vi "offload product.vi"   [LabVIEW 2023]
types:
  T1 = enum16{"plate1", "plate2", "plate3", "rinse", "seat"}
  T2 = enum16{"Initialize", "Absolute Position", "Relative Pickup", "Relative Dispense", "Swich valve", "Bypass"}
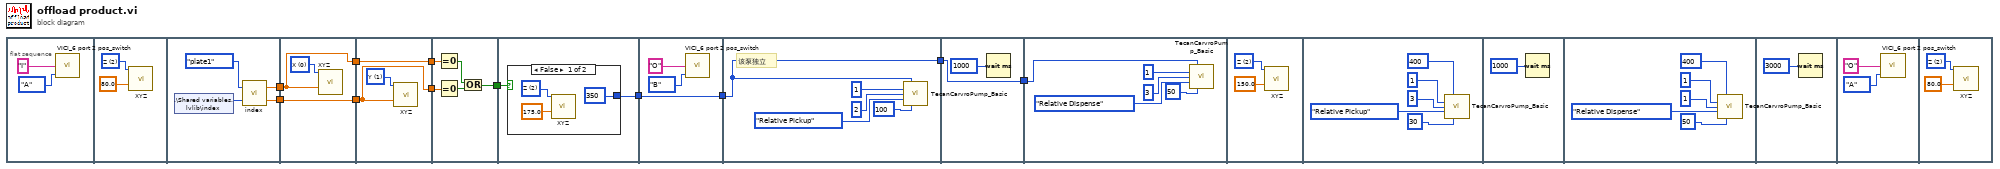
[diagram p0: block diagram]
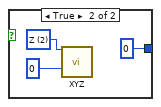
[diagram p2: hidden frame]
diagram:
  n1 = flat-sequence {
    tunnel: [w19] -> w11
    tunnel: [w18] -> w9
    tunnel: w11 -> [w20]
    tunnel: [w21] -> w10
    tunnel: w9 -> [w21]
    tunnel: [w20] -> w7
    tunnel: w10 -> [w23]
    tunnel: [w24] -> w8
    tunnel: w7 -> [w24]
    tunnel: [w23] -> w6
    tunnel: w8 -> [w30]
    tunnel: w6 -> [w29]
    tunnel: [w26] -> w5
    tunnel: w5 -> [w32]
    tunnel: [w31] -> w3
    tunnel: [w39] -> w4
    tunnel: w3 -> [w39]
    tunnel: w4 -> [w42]
    tunnel: [w42] -> w2
    tunnel: [w47] -> w1
    tunnel: w2 -> [w47]
    tunnel: w1 -> [w49]
    frame #0 {
      n2 = call "VICI_6 port 2 pos_switch.vi"("Switch to position (A/B)"=enum16{"A", "B"}."A", "Valve ID"="I") -> ()  [unwired: 2 in, 1 out]
    }
    frame #1 {
      w15 = u16 2 items=["X", "Y", "Z"] ("AXIS")
      n3 = call "XYZ.vi"("AXIS"=w15, "Set location (mm)"=80.0) -> ()  [unwired: 9 in, 5 out]
    }
    frame #2 {
      n4 = shared-variable ".\\Shared variables.lvlib\\index"() -> (w16:i8)  [unwired: 1 in, 1 out]
      n5 = call "index.vi"("index"=w16, "where"=T1."plate1") -> ("Y"=w18:dbl, "X"=w19:dbl)
    }
    frame #3 {
      w22 = u16 0 items=["X", "Y", "Z"] ("AXIS")
      n6 = call "XYZ.vi"("AXIS"=w22, "Set location (mm)"=w20) -> ()  [unwired: 9 in, 5 out]
    }
    frame #4 {
      w25 = u16 1 items=["X", "Y", "Z"] ("AXIS")
      n7 = call "XYZ.vi"("AXIS"=w25, "Set location (mm)"=w23) -> ()  [unwired: 9 in, 5 out]
    }
    frame #5 {
      n8 = Equal To 0?(x=w30) -> (x = 0?=w28:bool)
      n9 = Equal To 0?(x=w29) -> (x = 0?=w27:bool)
      n10 = Or(x=w28, y=w27) -> (x .or. y?=w26:bool)
    }
    frame #6 {
      n11 = case shown="False" w32 {
        tunnel: [u16 350 ("Volume (μL)") u16 0 ("Volume (μL)")] -> w31
        frame False {
          w35 = u16 2 items=["X", "Y", "Z"] ("AXIS")
          n12 = call "XYZ.vi"("AXIS"=w35, "Set location (mm)"=175.0) -> ()  [unwired: 9 in, 5 out]
        }
        frame True {
          w37 = u16 2 items=["X", "Y", "Z"] ("AXIS")
          n13 = call "XYZ.vi"("AXIS"=w37, "Set location (mm)"=0) -> ()  [unwired: 9 in, 5 out]
        }
      }
    }
    frame #7 {
      n14 = call "VICI_6 port 2 pos_switch.vi"("Switch to position (A/B)"=enum16{"A", "B"}."B", "Valve ID"="O") -> ()  [unwired: 2 in, 1 out]
    }
    frame #8 {
      # "该泵独立"
      n15 = call "TecanCarvroPump_Basic.vi"("Volume (μL)"=w42, "TecanPump address"=u8 1, "Valve"=u8 2, "Mode"=T2."Relative Pickup", "Speed (μL/s)"=u16 100) -> ()  [unwired: 10 in, 1 out]
    }
    frame #9 {
      n16 = Wait (ms)(milliseconds to wait=u32 1000) -> ()  [unwired: 1 out]
    }
    frame #10 {
      n17 = call "TecanCarvroPump_Basic.vi"("Volume (μL)"=w49, "TecanPump address"=u8 1, "Valve"=u8 3, "Mode"=T2."Relative Dispense", "Speed (μL/s)"=u16 50) -> ()  [unwired: 10 in, 1 out]
    }
    frame #11 {
      w55 = u16 2 items=["X", "Y", "Z"] ("AXIS")
      n18 = call "XYZ.vi"("AXIS"=w55, "Set location (mm)"=150.0) -> ()  [unwired: 9 in, 5 out]
    }
    frame #12 {
      n19 = call "TecanCarvroPump_Basic.vi"("Volume (μL)"=u16 400, "TecanPump address"=u8 1, "Valve"=u8 3, "Mode"=T2."Relative Pickup", "Speed (μL/s)"=u16 30) -> ()  [unwired: 10 in, 1 out]
    }
    frame #13 {
      n20 = Wait (ms)(milliseconds to wait=u32 1000) -> ()  [unwired: 1 out]
    }
    frame #14 {
      n21 = call "TecanCarvroPump_Basic.vi"("Volume (μL)"=u16 400, "TecanPump address"=u8 1, "Valve"=u8 1, "Mode"=T2."Relative Dispense", "Speed (μL/s)"=u16 50) -> ()  [unwired: 10 in, 1 out]
    }
    frame #15 {
      n22 = Wait (ms)(milliseconds to wait=u32 3000) -> ()  [unwired: 1 out]
    }
    frame #16 {
      n23 = call "VICI_6 port 2 pos_switch.vi"("Switch to position (A/B)"=enum16{"A", "B"}."A", "Valve ID"="O") -> ()  [unwired: 2 in, 1 out]
    }
    frame #17 {
      w71 = u16 2 items=["X", "Y", "Z"] ("AXIS")
      n24 = call "XYZ.vi"("AXIS"=w71, "Set location (mm)"=80.0) -> ()  [unwired: 9 in, 5 out]
    }
  }
